vi "VI Tree.vi"   [LabVIEW 2012, in "Phidget Capacitive Touch.lvlib"]
doc: "${CapacitiveTouch:VITreeHeader}"
uses:
  <instrlib>/Phidgets/Phidget Capacitive Touch/Phidget Capacitive Touch.lvlib
  <instrlib>/Phidgets/Phidget Capacitive Touch/Public/CapacitiveTouchStart.vi
  <instrlib>/Phidgets/Phidget Capacitive Touch/Public/CapacitiveTouchOpen.vi
  <instrlib>/Phidgets/Phidget Capacitive Touch/Public/CapacitiveTouchClose.vi
panel:
  # "(c) 2015 Phidgets Inc..  ALL RIGHTS RESERVED."
  # "SEE DIAGRAM\nFOR VI TREE."
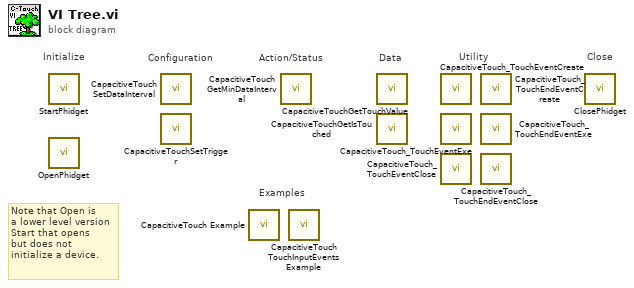
[diagram p0: block diagram]
diagram:
  # "Note that Open is\na lower level version\nStart that opens\nbut does not \ninitialize a device."
  # "Examples"
  # "Configuration"
  # "Utility"
  # "Data"
  # "Action/Status"
  # "Close"
  # "Initialize"
  n1 = call-poly <instrlib>:"StartPhidget.vi"() -> ()  [unwired: 12 in, 4 out]
  n2 = call-poly <instrlib>:"OpenPhidget.vi"() -> ()  [unwired: 8 in, 4 out]
  n3 = call <instrlib>:"CapacitiveTouchSetDataInterval.vi"() -> ()  [unwired: 9 in, 2 out]
  n4 = call <instrlib>:"CapacitiveTouchSetTrigger.vi"() -> ()  [unwired: 9 in, 2 out]
  n5 = call <instrlib>:"CapacitiveTouch Example.vi"() -> ()  [unwired: 12 in]
  n6 = call <instrlib>:"CapacitiveTouchGetMinDataInterval.vi"() -> ()  [unwired: 8 in, 3 out]
  n7 = call <instrlib>:"CapacitiveTouch TouchInputEvents Example.vi"() -> ()  [unwired: 12 in]
  n8 = call <instrlib>:"CapacitiveTouchGetTouchValue.vi"() -> ()  [unwired: 8 in, 3 out]
  n9 = call <instrlib>:"CapacitiveTouchGetIsTouched.vi"() -> ()  [unwired: 8 in, 3 out]
  n10 = call <instrlib>:"CapacitiveTouch_TouchEventCreate.vi"() -> ()  [unwired: 9 in, 3 out]
  n11 = call <instrlib>:"CapacitiveTouch_TouchEventExe.vi"() -> ()  [unwired: 5 in, 7 out]
  n12 = call <instrlib>:"CapacitiveTouch_TouchEventClose.vi"() -> ()  [unwired: 10 in, 2 out]
  n13 = call <instrlib>:"CapacitiveTouch_TouchEndEventCreate.vi"() -> ()  [unwired: 9 in, 3 out]
  n14 = call <instrlib>:"CapacitiveTouch_TouchEndEventExe.vi"() -> ()  [unwired: 6 in, 6 out]
  n15 = call <instrlib>:"CapacitiveTouch_TouchEndEventClose.vi"() -> ()  [unwired: 10 in, 2 out]
  n16 = call-poly <instrlib>:"ClosePhidget.vi"() -> ()  [unwired: 11 in, 1 out]
